vi "Calculate New Sector Location After Analysis.vi"(10 "2nd Analysis Sector":u8, 11 "Preanalysis Sector":u8) -> (3 "New Sector":u16)   [LabVIEW 2013]
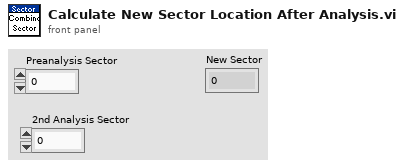
[diagram p1: front panel]
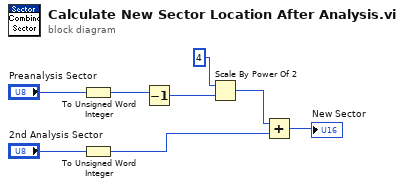
[diagram p0: block diagram]
diagram:
  n1 = To Unsigned Word Integer(number="Preanalysis Sector") -> (unsigned 16bit integer=w2:u16)
  n2 = To Unsigned Word Integer(number="2nd Analysis Sector") -> (unsigned 16bit integer=w1:u16)
  n3 = Decrement(x=w2) -> (x-1=w6:u16)
  n4 = Scale By Power Of 2(n=i16 4, x=w6) -> (x*2^n=w4:u16)
  n5 = Add(x=w4, y=w1) -> (x+y=→"New Sector":u16)
